vi "audio-stim2.vi"(11 "Stimulus List":dbl[][](array[numeric])=[[0.0, 3.0, 0.2, 1.0, 500.0], [1.0, 3.0, 0.2, 1.0, 500.0], [2.0, 3.0, 0.2, 1.0, 500.0], [3.0, 3.0, 0.2, 1.0, 1000.0], [4.0, 3.0, 0.2, 1.0, 500.0], [5.0, 3.0, 0.2, 1.0, 500.0], [6.0, 3.0, 0.2, 1.0, 1000.0], [7.0, 3.0, 0.2, 1.0, 1000.0], [8.0, 3.0, 0.2, 1.0, 1000.0], [9.0, 3.0, 0.2, 1.0, 500.0], [10.0, 3.0, 0.2, 1.0, 500.0], [11.0, 3.0, 0.2, 1.0, 1000.0], [12.0, 3.0, 0.2, 1.0, 1000.0], [13.0, 3.0, 0.2, 1.0, 1000.0], [14.0, 3.0, 0.2, 1.0, 1000.0], [15.0, 3.0, 0.2, 1.0, 1000.0], [16.0, 3.0, 0.2, 1.0, 500.0], [17.0, 3.0, 0.2, 1.0, 500.0], [18.0, 3.0, 0.2, 1.0, 500.0], [19.0, 3.0, 0.2, 1.0, 1000.0]]) -> (3 "Playing":bool=TRUE caption="Playing stimulus")   [LabVIEW 2013]
uses:
  <vilib>/DAQmx/write.llb/DAQmx Write (Digital U16 1Chan 1Samp).vi
  <vilib>/DAQmx/write.llb/DAQmx Write (Analog Wfm 1Chan NSamp).vi
  <vilib>/DAQmx/create/channels.llb/DAQmx Create Channel (AO-Voltage-Basic).vi
  <vilib>/DAQmx/create/channels.llb/DAQmx Create Channel (DO-Digital Output).vi
  <vilib>/DAQmx/miscellaneous.llb/DAQmx Fill In Error Info.vi
  <vilib>/DAQmx/configure/timing.llb/DAQmx Timing (Use Waveform).vi
panel:
  in  "Total Trials":i32=1 min=1 step=1
  out "Total Played":i32 caption="Total Played or Cued"
  in  "Save Stimulus List":bool
  in  "Load Stimulus List":bool
  out "Stimulus List Path":path
  out "Log File Path":path
  in  "Play Interval Jitter (s)":dbl=0.5
  in  "Play Interval (s)":dbl=1.0
  out "error out":errorcluster
  in  "DO Ports":tag="Dev1/port0:1" caption="DO Ports\n(\"browse\" and select two 8 bit ports)"
  in  "Sound AO Channel":tag="Dev1/ao0"
  out "Curr Param":dbl[](array[numeric])=[0.0, 3.0, 0.2, 1.0, 500.0] caption="Current (or Cued) Trial Parameters"
  in  "Sampling Rate":dbl=100000.0
  in  "stop":bool
  in  "Play":bool
  out "Current (or Cued) Waveform":waveform(dbl)(graph)={"t0"=timestamp(0 s since 1904-01-01), "dt"=1e-05, "Y"=array[19999 elements]}
  out "Waiting":bool=TRUE
  # "Stim#, Stim Type, Duration, Amplitude, Param 1, Param 2, Param 3, Param 4"
  # "Stim Type 1 DC (no parameters, just amplitude)"
  # "Stim Type 3 Pure Tone (param1 = frequency)"
  # "Stim Type 4 FM Sweep (param1 = start frequency, param2 = end frequency)"
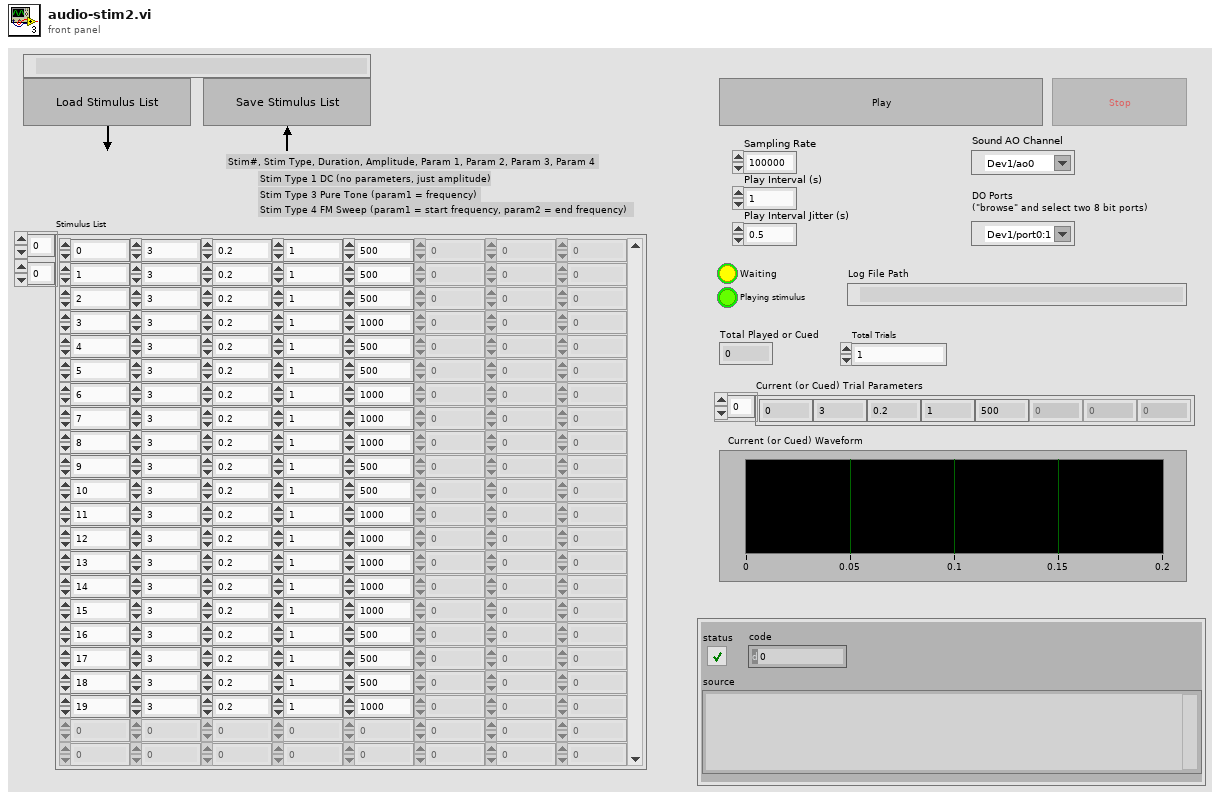
[diagram p1: front panel]
types:
  T1 = enum8{"Enabled", "Disabled", "Disabled and Grayed Out"}
  T2 = cluster{"Sampling Rate":dbl, "Value 3":dbl, dbl, "Value 2":dbl}
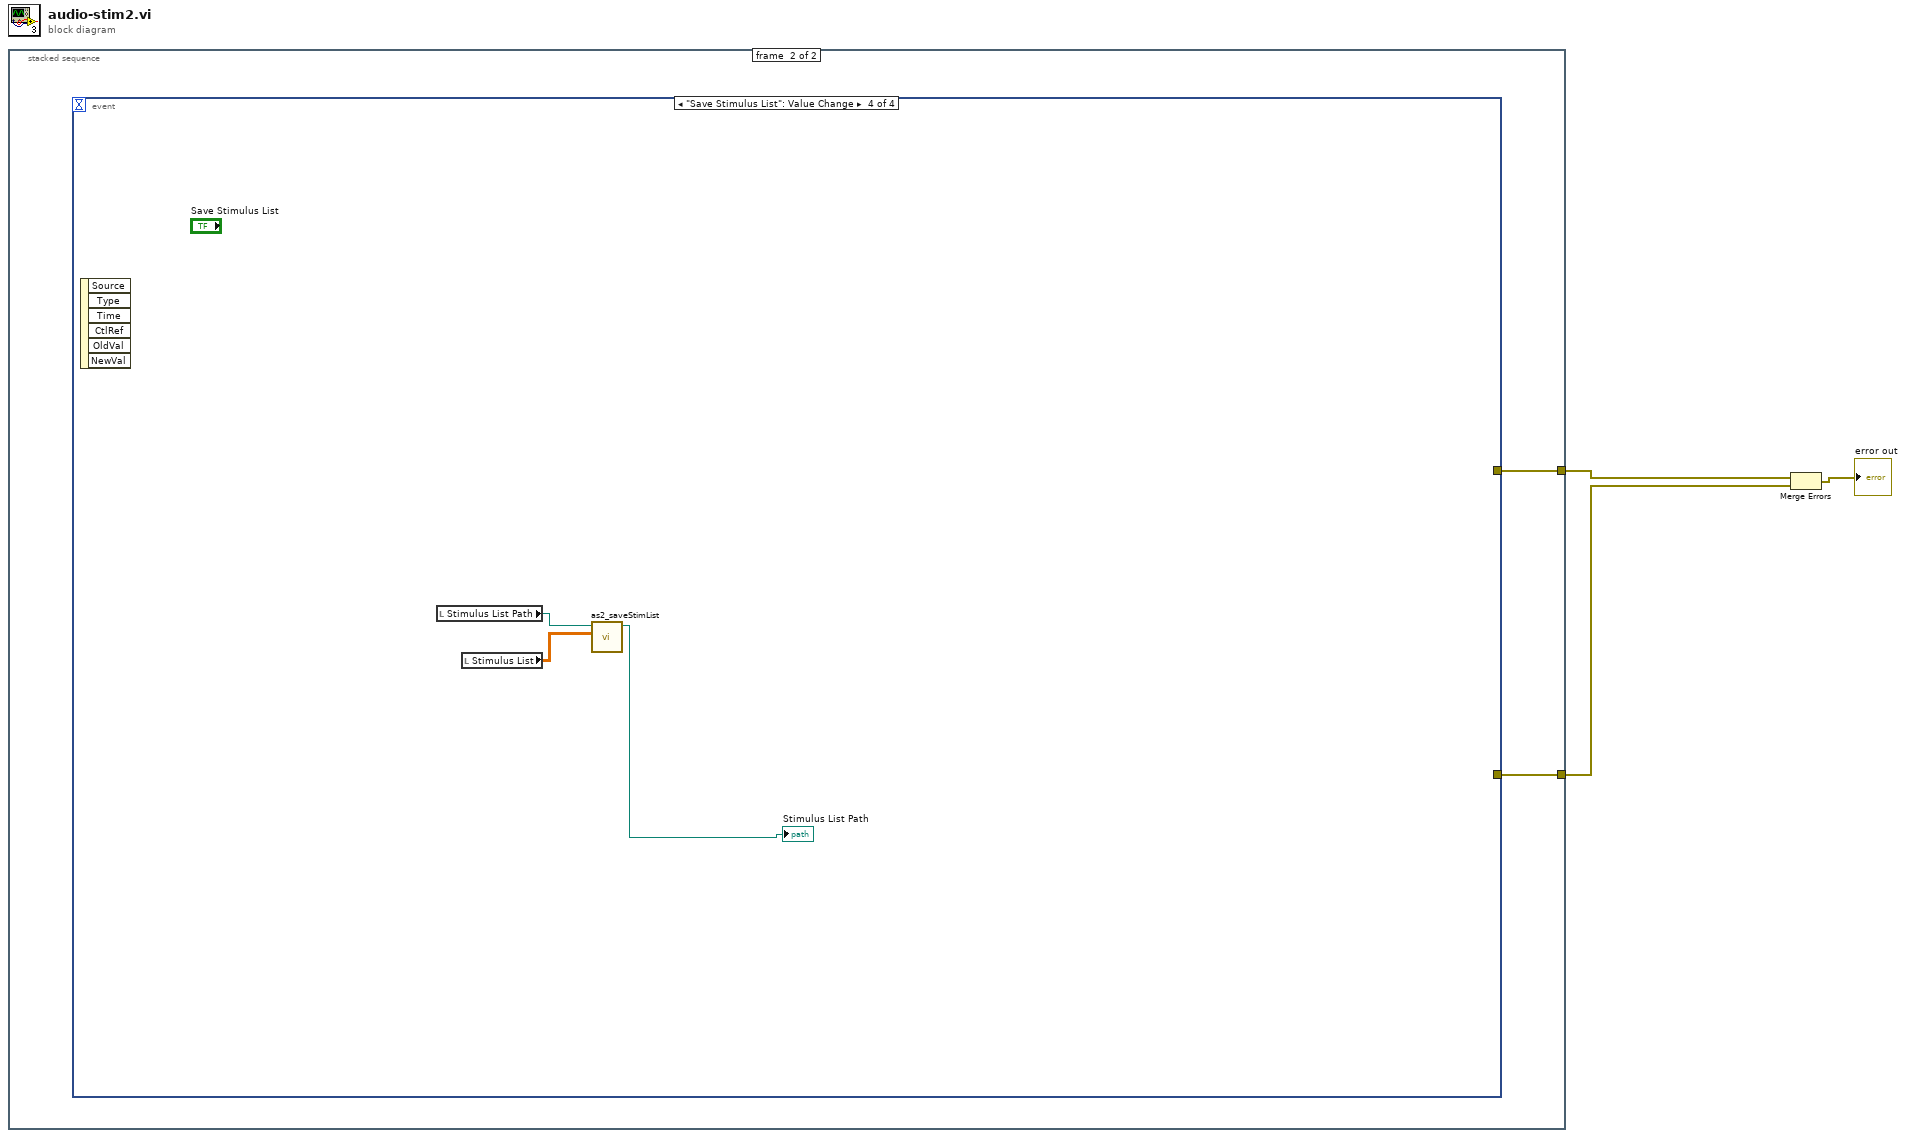
[diagram p0: block diagram]
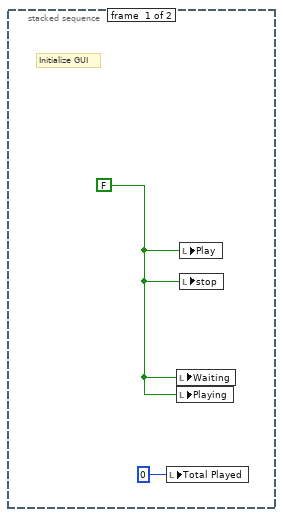
[diagram p2: hidden frame]
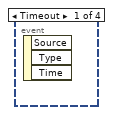
[diagram p3: hidden frame]
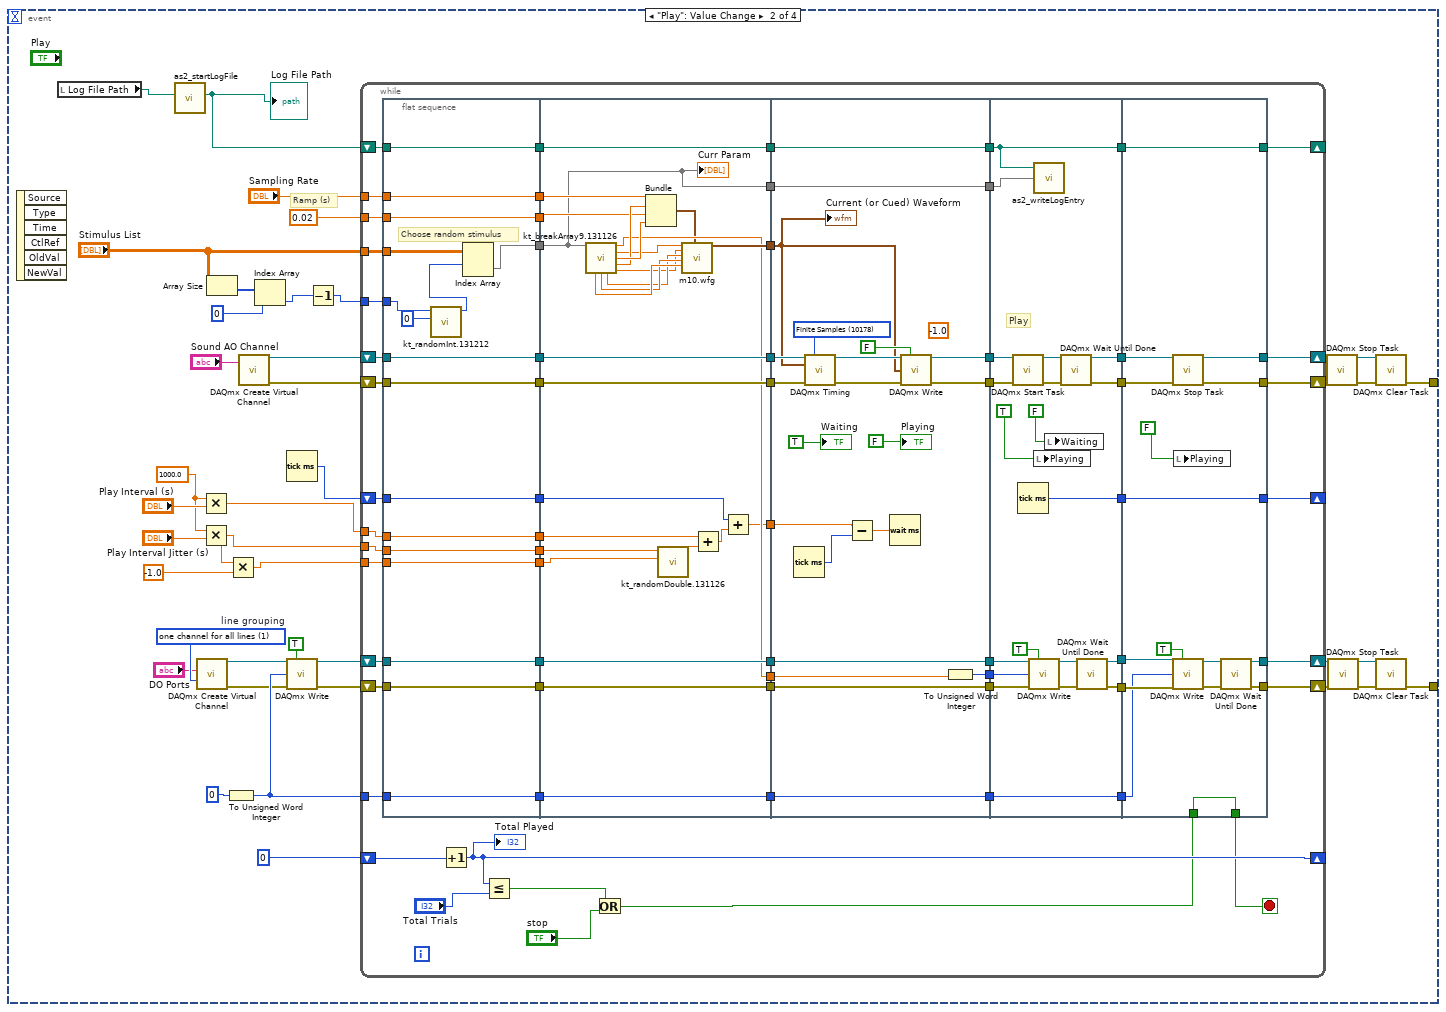
[diagram p4: hidden frame]
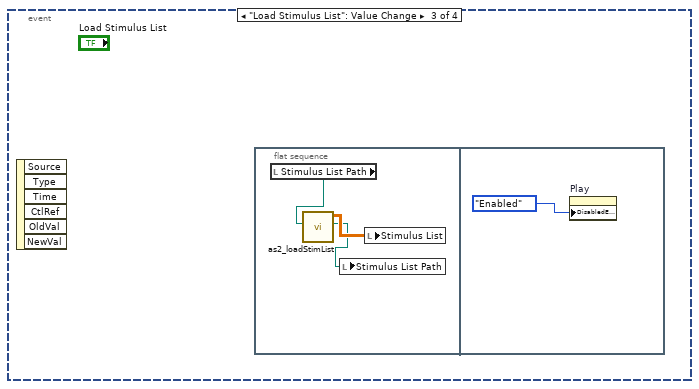
[diagram p5: hidden frame]
diagram:
  n1 = stacked-sequence {
    tunnel: [_ w7] -> w3
    tunnel: [_ w6] -> w2
    frame #0 {
      w5 = FALSE ("Play")
      # "Initialize GUI"
      n2 = local write "Total Played"(0 ("Total Played")) -> ()
      n3 = local write "Waiting"(w5) -> ()
      n4 = local write "Playing"(w5) -> ()
      n5 = local write "Play"(w5) -> ()
      n6 = local write "stop"(w5) -> ()
    }
    frame #1 {
      n7 = event shown="[3] \"Save Stimulus List\": Value Change" {
        selector: _ -> [_ _ _ _]
        dyn-events: _ -> [_ _ _ _]
        timeout: _ -> [_ _ _ _]
        tunnel: [_ w24 _ _] -> w7
        tunnel: [_ w23 _ _] -> w6
        event Timeout {
          n8 = event-data() -> ()  [unwired: 1 in, 3 out]
        }
        event "Play": Value Change {
          w17 = 1000.0 ("y")
          w44 = 1 items=["one channel for each line", "one channel for all lines"]  # line grouping
          # "Ramp (s)"
          n9 = event-data() -> ()  [unwired: 1 in, 6 out]
          n10 = local read "Log File Path"() -> (w12:path)
          n11 = call "as2_startLogFile.vi"("Path In"=w12) -> ("Path"=w11:path)  [unwired: 5 in, 1 out]
          "Log File Path" <- w11
          n12 = call-poly <vilib>:"DAQmx Create Virtual Channel.vi"("lines"="DO Ports", "line grouping"=w44) -> ("task out"=w22:refnum<k21>, "error out"=w21:errorcluster)  [unwired: 12 in]
          n13 = Multiply(x=w17, y="Play Interval (s)") -> (x*y=w16:dbl)
          n14 = Multiply(x=w17, y="Play Interval Jitter (s)") -> (x*y=w14:dbl)
          n15 = Array Size(array="Stimulus List") -> (size(s)=w42:i32[])
          n16 = To Unsigned Word Integer(number=u16 0 ("data")) -> (unsigned 16bit integer=w27:u16)
          n17 = Multiply(x=w14, y=-1.0) -> (x*y=w15:dbl)
          n18 = call-poly <vilib>:"DAQmx Create Virtual Channel.vi"("physical channels"="Sound AO Channel") -> ("task out"=w26:refnum<k21>, "error out"=w25:errorcluster)  [unwired: 13 in]
          n19 = Index Array(array=w42, index=0) -> (element=w10:i32)
          n20 = Tick Count (ms)() -> (millisecond timer value=w13:u32)
          n21 = call-poly <vilib>:"DAQmx Write.vi"("task/channels in"=w22, "auto start"=TRUE, "data"=w27, "error in"=w21) -> ("task out"=w31:refnum<k21>, "error out"=w30:errorcluster)  [unwired: 9 in, 1 out]
          n22 = Decrement(x=w10) -> (x-1=w9:i32)
          n23 = while {
            tunnel: "Stimulus List" -> [w85]
            tunnel: "Sampling Rate" -> [w84]
            tunnel: 0.02 -> [w83]
            shift-right: [w110] -> w36
            shift-left: w26 -> [w108]
            shift-right: [w109] -> w35
            shift-left: w25 -> [w107]
            shift-right: [w99] -> w40
            shift-left: w31 -> [w106]
            shift-right: [w98] -> w39
            shift-left: w30 -> [w93]
            shift-right: [w51] -> _
            shift-left: 0 ("data") -> [w52]
            tunnel: w27 -> [w96]
            shift-right: [w80] -> _
            shift-left: w13 -> [w79]
            tunnel: w16 -> [w75]
            tunnel: w15 -> [w76]
            tunnel: w14 -> [w77]
            shift-right: [w68] -> _
            shift-left: w11 -> [w74]
            tunnel: w9 -> [w54]
            stop <- w49 stop-if-true
            n24 = flat-sequence {
              tunnel: w74 -> [w118]
              tunnel: w75 -> [w119]
              tunnel: w76 -> [w120]
              tunnel: w77 -> [w121]
              tunnel: w79 -> [w122]
              tunnel: w83 -> [w123]
              tunnel: w84 -> [w124]
              tunnel: w85 -> [w115]
              tunnel: w93 -> [w125]
              tunnel: w96 -> [w126]
              tunnel: w106 -> [w127]
              tunnel: w107 -> [w128]
              tunnel: w108 -> [w129]
              tunnel: [w129] -> w67
              tunnel: [w128] -> w66
              tunnel: [w127] -> w65
              tunnel: [w126] -> w64
              tunnel: [w125] -> w63
              tunnel: [w113] -> w62
              tunnel: [w124] -> w61
              tunnel: [w123] -> w60
              tunnel: [w122] -> w59
              tunnel: [w121] -> w58
              tunnel: [w120] -> w57
              tunnel: [w119] -> w56
              tunnel: [w118] -> w55
              tunnel: w54 -> [w117]
              tunnel: [w155] -> w91
              tunnel: [w154] -> w90
              tunnel: [w153] -> w89
              tunnel: [w152] -> w88
              tunnel: [w151] -> w87
              tunnel: [w143] -> w86
              tunnel: [w140] -> w82
              tunnel: [w137] -> w78
              tunnel: [w131] -> w73
              tunnel: [w130] -> w72
              tunnel: w67 -> [w155]
              tunnel: w66 -> [w154]
              tunnel: w65 -> [w153]
              tunnel: w64 -> [w152]
              tunnel: w63 -> [w151]
              tunnel: w62 -> [w130]
              tunnel: w61 -> [w142]
              tunnel: w60 -> [w141]
              tunnel: w59 -> [w138]
              tunnel: w58 -> [w136]
              tunnel: w57 -> [w135]
              tunnel: w56 -> [w132]
              tunnel: w55 -> [w131]
              tunnel: [w166] -> w112
              tunnel: [w165] -> w111
              tunnel: [w175] -> w105
              tunnel: [w174] -> w100
              tunnel: [w173] -> w97
              tunnel: [w163] -> w92
              tunnel: w91 -> [w172]
              tunnel: w90 -> [w171]
              tunnel: w89 -> [w175]
              tunnel: w88 -> [w173]
              tunnel: w87 -> [w163]
              tunnel: w86 -> [w162]
              tunnel: w82 -> [w161]
              tunnel: w78 -> [w158]
              tunnel: w73 -> [w156]
              tunnel: w72 -> [w157]
              tunnel: [w157] -> w71
              tunnel: [w156] -> w70
              tunnel: w112 -> [w186]
              tunnel: w111 -> [w185]
              tunnel: w105 -> [w194]
              tunnel: [w188] -> w104
              tunnel: [w187] -> w103
              tunnel: [w191] -> w102
              tunnel: [w190] -> w101
              tunnel: w100 -> [w195]
              tunnel: w97 -> [w189]
              tunnel: [w189] -> w95
              tunnel: w92 -> [w180]
              tunnel: [w179] -> w81
              tunnel: w71 -> [w178]
              tunnel: w70 -> [w177]
              tunnel: [w177] -> w69
              tunnel: [w200] -> w109
              tunnel: [w201] -> w110
              tunnel: w104 -> [w203]
              tunnel: w103 -> [w202]
              tunnel: w102 -> [w211]
              tunnel: w101 -> [w210]
              tunnel: [w206] -> w99
              tunnel: [w205] -> w98
              tunnel: w95 -> [w204]
              tunnel: w81 -> [w199]
              tunnel: [w199] -> w80
              tunnel: w69 -> [w198]
              tunnel: [w198] -> w68
              tunnel: w50 -> [w197]
              tunnel: [w197] -> w49
              frame #0 {
                # "Choose random stimulus"
                n25 = call "kt_randomInt.131212.vi"("Min"=0, "Max"=w117) -> ("Random"=w114:i32)  [unwired: 9 in]
                n26 = Index Array(array=w115, index (row)=w114) -> (element=w113:dbl[])  [unwired: 1 in]
              }
              frame #1 {
                n27 = call "kt_breakArray9.131126.vi"("Current (or Cued Trial Parameters)"=w130) -> ("Value 0"=w140:dbl, "Value 1"=w144:dbl, "Value 2"=w146:dbl, "Value 3"=w145:dbl, "Value 7"=w150:dbl, "Value 6"=w149:dbl, "Value 5"=w148:dbl, "Value 4"=w147:dbl)  [unwired: 6 in, 1 out]
                n28 = Bundle("Sampling Rate"=w142, "Value 3"=w145, w141, "Value 2"=w146) -> (w139:T2)  [unwired: 1 in]
                n29 = call "kt_randomDouble.131126.vi"("Min"=w135, "Max"=w136) -> ("Random"=w133:dbl)  [unwired: 9 in]
                n30 = call "m10.wfg.vi"("Stimulus Type"=w144, "Param 0"=w147, "Param 1"=w148, "Param 2"=w149, "Param 3"=w150, "Waveform Properties"=w139) -> ("Waveform Out"=w143:waveform(dbl))  [unwired: 12 in, 1 out]
                n31 = Add(x=w132, y=w133) -> (x+y=w134:dbl)
                n32 = Add(x=w138, y=w134) -> (x+y=w137:dbl)
                "Curr Param" <- w130
              }
              frame #2 {
                (unwired) -1.0 ("timeout")
                w170 = 10178 items=["Finite Samples"=10178, "Continuous Samples"=10123, "Hardware Timed Single Point"=12522] ("sample mode")
                n33 = Tick Count (ms)() -> (millisecond timer value=w159:u32)
                n34 = call-poly <vilib>:"DAQmx Timing.vi"("task/channels in"=w172, "sample mode"=w170, "waveform"=w162, "error in"=w171) -> ("task out"=w169:refnum<k21>, "error out"=w168:errorcluster)  [unwired: 10 in]
                n35 = Subtract(x=w158, y=w159) -> (x-y=w160:dbl)
                n36 = Wait (ms)(milliseconds to wait=w160) -> ()  [unwired: 1 out]
                n37 = call-poly <vilib>:"DAQmx Write.vi"("task/channels in"=w169, "auto start"=FALSE, "data"=w162, "error in"=w168) -> ("task out"=w166:refnum<k21>, "error out"=w165:errorcluster)  [unwired: 9 in, 1 out]
                n38 = To Unsigned Word Integer(number=w161) -> (unsigned 16bit integer=w174:u16)
                "Waiting" <- TRUE ("Playing Stimulus")
                "Playing" <- FALSE ("Playing Stimulus")
                "Current (or Cued) Waveform" <- w162
              }
              frame #3 {
                # "Play"
                n39 = call <vilib>:"DAQmx Start Task.vi"("task/channels in"=w186, "error in"=w185) -> ("task out"=w184:refnum<k21>, "error out"=w183:errorcluster)  [unwired: 12 in]
                n40 = Tick Count (ms)() -> (millisecond timer value=w179:u32)
                n41 = call-poly <vilib>:"DAQmx Write.vi"("task/channels in"=w194, "auto start"=TRUE, "data"=w195, "error in"=w180) -> ("task out"=w193:refnum<k21>, "error out"=w192:errorcluster)  [unwired: 9 in, 1 out]
                n42 = call "as2_writeLogEntry.vi"("Path In"=w177, "Curr Param"=w178) -> ()  [unwired: 4 in, 1 out]
                n43 = local write "Playing"(TRUE ("Playing Stimulus")) -> ()
                n44 = local write "Waiting"(FALSE ("Playing Stimulus")) -> ()
                n45 = call <vilib>:"DAQmx Wait Until Done.vi"("task/channels in"=w184, "error in"=w183) -> ("task out"=w188:refnum<k21>, "error out"=w187:errorcluster)  [unwired: 12 in]
                n46 = call <vilib>:"DAQmx Wait Until Done.vi"("task/channels in"=w193, "error in"=w192) -> ("task out"=w191:refnum<k21>, "error out"=w190:errorcluster)  [unwired: 12 in]
              }
              frame #4 {
                n47 = call <vilib>:"DAQmx Stop Task.vi"("task/channels in"=w203, "error in"=w202) -> ("task out"=w201:refnum<k21>, "error out"=w200:errorcluster)  [unwired: 12 in]
                n48 = call-poly <vilib>:"DAQmx Write.vi"("task/channels in"=w211, "auto start"=TRUE, "data"=w204, "error in"=w210) -> ("task out"=w208:refnum<k21>, "error out"=w207:errorcluster)  [unwired: 9 in, 1 out]
                n49 = local write "Playing"(FALSE ("Playing Stimulus")) -> ()
                n50 = call <vilib>:"DAQmx Wait Until Done.vi"("task/channels in"=w208, "error in"=w207) -> ("task out"=w206:refnum<k21>, "error out"=w205:errorcluster)  [unwired: 12 in]
              }
            }
            n51 = Increment(x=w52) -> (x+1=w51:i32)
            "Total Played" <- w51
            n52 = Less Or Equal?(x=w51, y="Total Trials") -> (x <= y?=w94:bool)
            n53 = Or(x=w94, y="stop") -> (x .or. y?=w50:bool)
          }
          n54 = call <vilib>:"DAQmx Stop Task.vi"("task/channels in"=w36, "error in"=w35) -> ("task out"=w34:refnum<k21>, "error out"=w33:errorcluster)  [unwired: 12 in]
          n55 = call <vilib>:"DAQmx Stop Task.vi"("task/channels in"=w40, "error in"=w39) -> ("task out"=w38:refnum<k21>, "error out"=w37:errorcluster)  [unwired: 12 in]
          n56 = call <vilib>:"DAQmx Clear Task.vi"("task in"=w34, "error in"=w33) -> ("error out"=w24:errorcluster)  [unwired: 13 in]
          n57 = call <vilib>:"DAQmx Clear Task.vi"("task in"=w38, "error in"=w37) -> ("error out"=w23:errorcluster)  [unwired: 13 in]
        }
        event "Load Stimulus List": Value Change {
          n58 = event-data() -> ()  [unwired: 1 in, 6 out]
          n59 = flat-sequence {
            frame #0 {
              n60 = local read "Stimulus List Path"() -> (w215:path)
              n61 = call "as2_loadStimList.vi"("Path In"=w215) -> ("Path"=w213:path, "Stimulus List"=w214:dbl[][])  [unwired: 4 in, 1 out]
              n62 = local write "Stimulus List Path"(w213) -> ()
              n63 = local write "Stimulus List"(w214) -> ()
            }
            frame #1 {
              n64 = property on="Play" class="Bool (strict)"("DisabledEnum"=T1."Enabled" ("Disabled")) -> ()  [unwired: 2 in, 2 out]
            }
          }
        }
        event "Save Stimulus List": Value Change {
          n65 = event-data() -> ()  [unwired: 1 in, 6 out]
          n66 = local read "Stimulus List Path"() -> (w219:path)
          n67 = local read "Stimulus List"() -> (w218:dbl[][])
          n68 = call "as2_saveStimList.vi"("Stimulus List"=w218, "Path In"=w219) -> ("Path"=→"Stimulus List Path":path)  [unwired: 4 in, 1 out]
        }
      }
    }
  }
  n69 = Merge Errors(w3, w2) -> (→"error out":errorcluster)
